vi "Spartan HTTP Config Loader.vi"(4 "error in (no error)":errorcluster, 7 "lvhttp.cfg":path=path "") -> (0 "error out":errorcluster, 3 "Config Load Message":string)   [LabVIEW 2011]
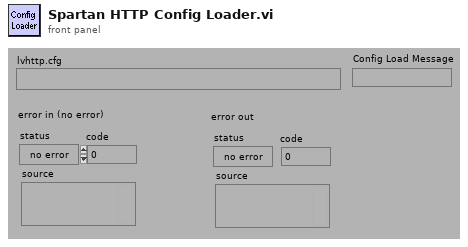
[diagram p1: front panel]
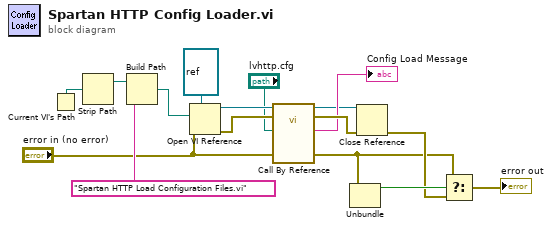
[diagram p0: block diagram]
diagram:
  n1 = Current VI's Path() -> (path=w9:path)
  n2 = Strip Path(path=w9) -> (stripped path=w10:path)  [unwired: 1 out]
  n3 = Build Path(base path=w10, name or relative path="Spartan HTTP Load Configuration Files.vi") -> (appended path=w12:path)
  n4 = Open VI Reference(type specifier VI Refnum (for type only)=refnum<vi> refnum ("load config files"), vi path=w12, error in (no error)="error in (no error)") -> (vi reference=w6:refnum<vi>, error out=w8:errorcluster)  [unwired: 1 in, 2 out]
  n5 = call-by-ref "?"(reference=w6, error in=w8, 4:"error in"="error in (no error)", "lvhttp.cfg"="lvhttp.cfg") -> (reference out=w1:refnum<vi>, error out=w7:errorcluster, 0:"error out"=w4:errorcluster, "Config Load Message"=→"Config Load Message":string)  [unwired: 4 in]
  n6 = Unbundle(w4) -> ("status"=w15:bool)  [unwired: 2 out]
  n7 = Close Reference(reference=w1, error in (no error)=w7) -> (error out=w14:errorcluster)
  n8 = Select(t=w4, s=w15, f=w14) -> (s? t:f=→"error out":errorcluster)
